vi "FGV.vi"(7 "Enum":T1, 8 "error in (no error)":errorcluster, 10 "Array":u32[](array[numeric])) -> (0 "error out":errorcluster, 2 "Array 2":u32[](array[numeric]))   [LabVIEW 2013]
doc: "This subVI set the data and extract the data."
uses:
  Controls/FGV.ctl
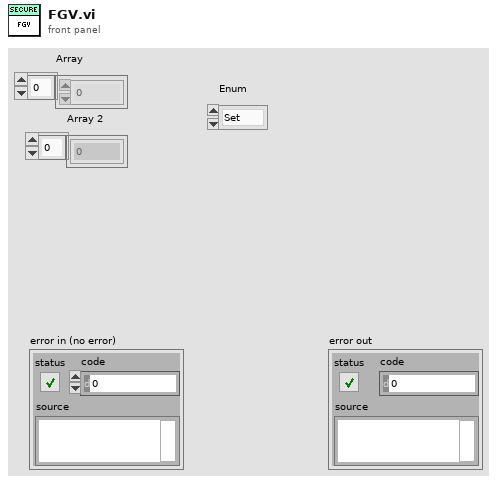
[diagram p1: front panel]
types:
  T1 = typedef "FGV.ctl" = enum16{"Set", "Get"}
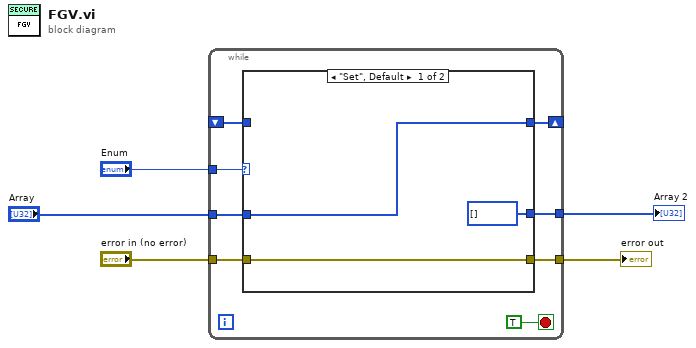
[diagram p0: block diagram]
diagram:
  n1 = while {
    tunnel: "Enum" -> [w13]
    tunnel: "Array" -> [w12]
    shift-right: [w11] -> _
    shift-left: _ -> [w10]
    tunnel: [w9] -> w1
    tunnel: "error in (no error)" -> [w7]
    tunnel: [w6] -> w5
    stop <- TRUE stop-if-true
    n2 = case shown="\"Set\", Default" w13 {
      tunnel: w12 -> [w16 _]
      tunnel: [w16 w18] -> w11
      tunnel: w10 -> [_ w18]
      tunnel: [i32[] [] ("Array") w18] -> w9
      tunnel: w7 -> [w15 w17]
      tunnel: [w15 w17] -> w6
      frame "Set", Default {
      }
      frame "Get" {
      }
    }
  }
  "error out" <- w5
  "Array 2" <- w1
